vi "LevelProbeInit.vi"() -> (0 "error out":errorcluster, 2 "read buffer":string, 3 "VISA resource name out":refnum<visa-resource-name>)   [LabVIEW 2018]
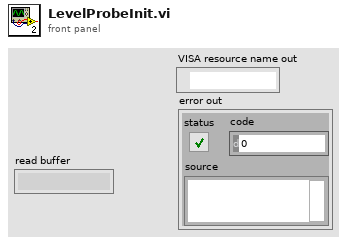
[diagram p1: front panel]
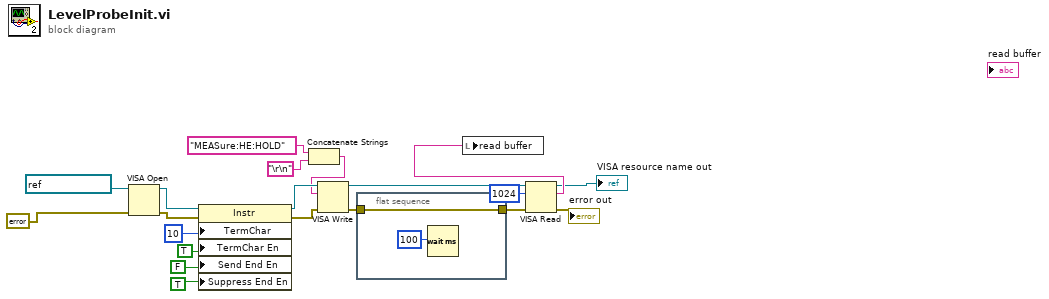
[diagram p0: block diagram]
diagram:
  n1 = VISA Open(error in (no error)=errorcluster {"status"=FALSE, "code"=0, "source"=""}, VISA resource name=refnum<visa-resource-name> "LevelProbe") -> (VISA resource name=w16:refnum<visa-resource-name>, error out=w15:errorcluster)  [unwired: 3 in]
  n2 = property class="Instr"(reference=w16, error in=w15, "TermChar"=u8 10 ("Message Based Settings:Termination Character"), "TermChar En"=TRUE ("Message Based Settings:Termination Character Enable"), "Send End En"=FALSE ("Message Based Settings:Send End Enable"), "Suppress End En"=TRUE ("Message Based Settings:Suppress End Enable")) -> (reference out=w13:refnum<visa-resource-name>, error out=w12:errorcluster)
  n3 = Concatenate Strings("MEASure:HE:HOLD" ("Command"), "\r\n") -> (w4:string)
  n4 = VISA Write(VISA resource name=w13, write buffer=w4, error in (no error)=w12) -> (VISA resource name out=w9:refnum<visa-resource-name>, error out=w11:errorcluster)  [unwired: 1 out]
  n5 = flat-sequence {
    tunnel: w11 -> [w21]
    tunnel: [w21] -> w10
    frame #0 {
      n6 = Wait (ms)(milliseconds to wait=100) -> ()  [unwired: 1 out]
    }
  }
  n7 = VISA Read(VISA resource name=w9, byte count=u32 1024, error in (no error)=w10) -> (VISA resource name out=→"VISA resource name out":refnum<visa-resource-name>, read buffer=w7:string, error out=→"error out":errorcluster)  [unwired: 1 out]
  n8 = local write "read buffer"(w7) -> ()
